vi "RefreshTimerFGV.vi"(7 "Command":enum16{"Initialize", "Check Time", "Reset"}(ring), 8 "Error In":errorcluster, 10 "Ticker Multiplier":dbl=10.0 format="%#_13g", 11 "Refresh Period [s]":dbl=5.0 format="%#_13g") -> (0 "Error Out":errorcluster, 2 "Time to Next Refresh":dbl, 3 "Refresh Now?":bool)   [LabVIEW 2017, in "Client.lvlib" / "CommsServer.lvlib"]
uses:
  CommsServer.lvlib
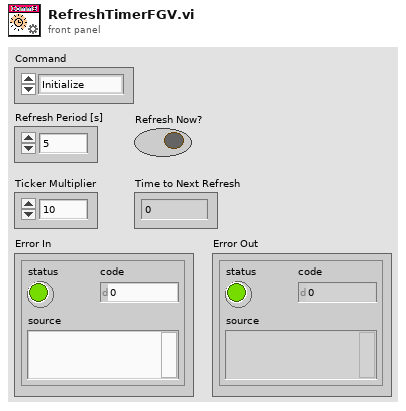
[diagram p1: front panel]
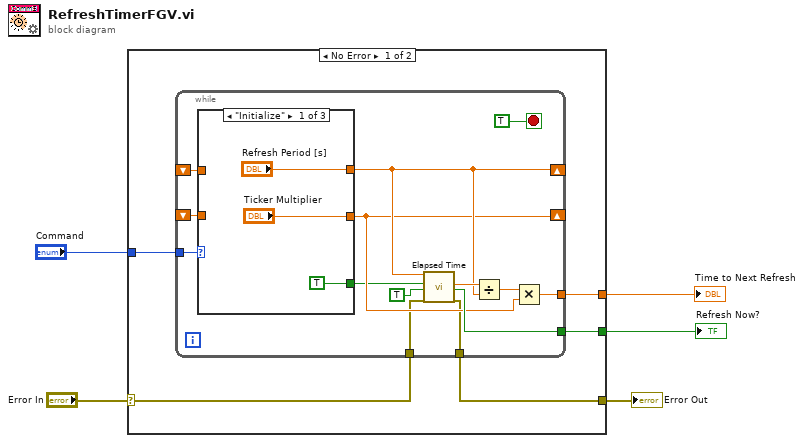
[diagram p0: block diagram]
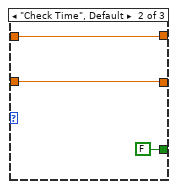
[diagram p2: hidden frame]
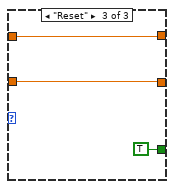
[diagram p3: hidden frame]
diagram:
  n1 = case shown="No Error" "Error In" {
    selector: "Error In" -> [w7 w34]
    tunnel: [w10 _] -> w5
    tunnel: [w9 _] -> w4
    tunnel: "Command" -> [w8 _]
    tunnel: [w6 w34] -> w1
    frame No Error {
      n2 = while {
        tunnel: [w24] -> w10
        tunnel: [w23] -> w9
        shift-right: [w19] -> _
        shift-left: _ -> [w16]
        shift-right: [w18] -> _
        shift-left: _ -> [w15]
        tunnel: w8 -> [w17]
        tunnel: w7 -> [w12]
        tunnel: [w11] -> w6
        stop <- TRUE stop-if-true
        n3 = case shown="\"Initialize\"" w17 {
          tunnel: ["Refresh Period [s]" w30 w33] -> w19
          tunnel: ["Ticker Multiplier" w29 w32] -> w18
          tunnel: w16 -> [_ w30 w33]
          tunnel: w15 -> [_ w29 w32]
          tunnel: [TRUE FALSE TRUE] -> w14
          frame "Initialize" {
          }
          frame "Check Time", Default {
          }
          frame "Reset" {
          }
        }
        n4 = call "Elapsed Time"("Time Target (s)"=w19, "Reset"=w14, "Auto Reset"=TRUE, "error in (no error)"=w12) -> ("Elapsed Time (s)"=w21:dbl, "Time has Elapsed"=w24:bool, "error out"=w11:errorcluster)  [unwired: 8 in, 5 out]
        n5 = Divide(x=w21, y=w19) -> (x/y=w20:dbl)
        n6 = Multiply(x=w20, y=w18) -> (x*y=w23:dbl)
      }
    }
    frame Error {
    }
  }
  "Refresh Now?" <- w5
  "Time to Next Refresh" <- w4
  "Error Out" <- w1
